vi "clearError.vi"(8 "error in (no error)":errorcluster, 10 "model":refnum<class "Model.lvclass">, 11 "FaultState in":refnum<class "FaultState.lvclass">) -> (0 "error out":errorcluster, 2 "model 2":refnum<class "Model.lvclass">, 3 "FaultState out":refnum<class "FaultState.lvclass">)   [LabVIEW 2013, in "FaultState.lvclass"]
uses:
  FaultState.lvclass
  Model/Model/Model.lvclass
  Typedefs/StateSelector.ctl
  Typedefs/M2AADTTypedefs.lvlib
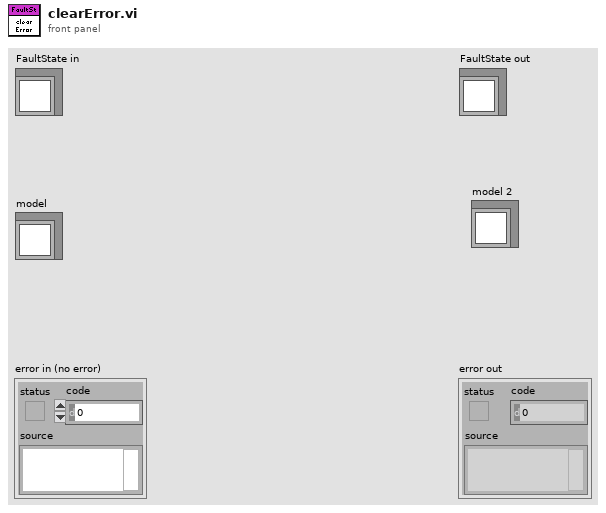
[diagram p1: front panel]
types:
  T1 = typedef "M2AADTTypedefs.lvlib/StateSelector.ctl" = enum16{"EndingCycleState", "FaultState", "InteractiveMotionState", "MovingToNewForceState", "OffState", "PausingState", "StandbyState", "StoppedState"}
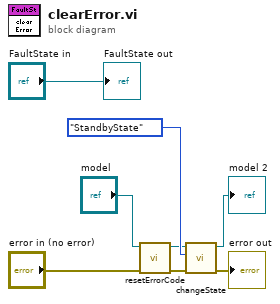
[diagram p0: block diagram]
diagram:
  n1 = call "resetErrorCode.vi"("error in (no error)"="error in (no error)", "Model in"="model") -> ("error out"=w2:errorcluster, "Model out"=w3:refnum<class "Model.lvclass">)  [unwired: 8 in]
  n2 = call "changeState.vi"("error in (no error)"=w2, "State:"=StateSelector."StandbyState", "Model in"=w3) -> ("error out"=→"error out":errorcluster, "Model out"=→"model 2":refnum<class "Model.lvclass">)  [unwired: 7 in]
  "FaultState out" <- "FaultState in"
